vi "Create Cree Communications.vi"(8 "error in (no error)":errorcluster, 9 "Comm Instrument":refnum<class "Comm Instrument.lvclass">, 10 "Position":u32, 11 "Calibration in":refnum<class "Calibration.lvclass">) -> (0 "error out":errorcluster, 2 "Cree Communications":refnum<class "Cree Communications.lvclass">, 3 "Calibration out":refnum<class "Calibration.lvclass">)   [LabVIEW 2015, in "Calibration.lvclass"]
uses:
  Calibration.lvclass
  Classes/Cree Communications/Class/Cree Communications.lvclass
  Classes/Instruments/Comm Instrument/Class/Comm Instrument.lvclass
  <vilib>/Cree, Inc/Cree Test Framework/Classes/Base Objects/Base Class/Base Class/Base Class.lvclass
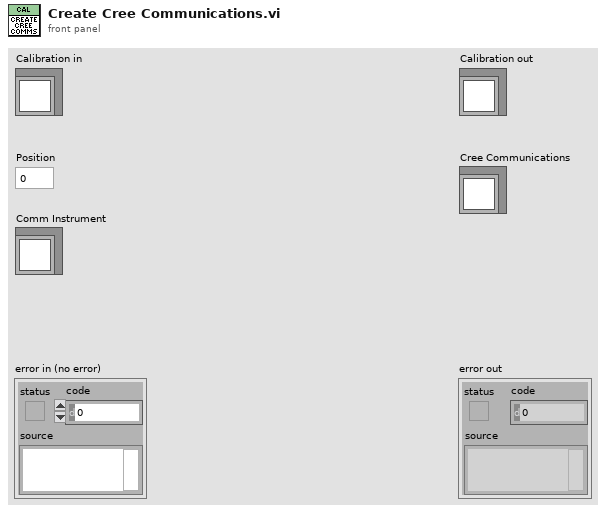
[diagram p1: front panel]
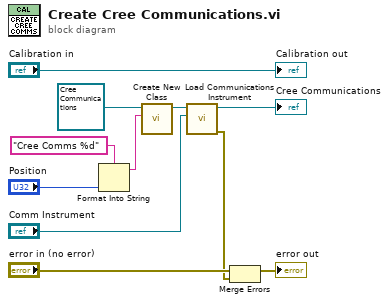
[diagram p0: block diagram]
diagram:
  n1 = Format Into String(format string="Cree Comms %d", "Position") -> (resulting string=w6:string)  [unwired: 2 in, 1 out]
  n2 = call <vilib>:"Create New Class.vi"("Name"=w6, "Base Class in"=refnum<class "Cree Communications.lvclass"> refnum ("Cree Communications")) -> ("Base Class out"=w5:refnum<class "Cree Communications.lvclass">)  [unwired: 8 in, 1 out]
  n3 = call "Load Communications Instrument.vi"("Communication Instrument"="Comm Instrument", "Cree Communications in"=w5) -> ("error out"=w1:errorcluster, "Cree Communications out"=→"Cree Communications":refnum<class "Cree Communications.lvclass">)  [unwired: 8 in]
  n4 = Merge Errors("error in (no error)", w1) -> (→"error out":errorcluster)
  "Calibration out" <- "Calibration in"
